vi "Get Control Values.vi"(8 "error in (no error)":errorcluster, 11 "Simulated Game Pad Interface in":refnum<class "Simulated Game Pad Interface.lvclass">) -> (0 "error out":errorcluster, 2 "Cluster":T1, 3 "Simulated Game Pad Interface out":refnum<class "Simulated Game Pad Interface.lvclass">)   [LabVIEW 2017, in "Simulated Game Pad Interface.lvclass"]
uses:
  Simulated Game Pad Interface.lvclass
  Abstract Game Pad Interface/Game Pad Descriptor.ctl
  Abstract Game Pad Interface/Abstract Game Pad Interface.lvclass
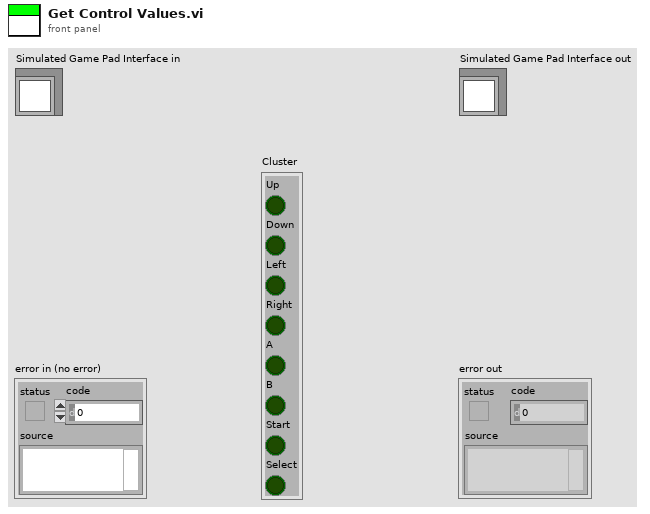
[diagram p1: front panel]
types:
  T1 = typedef "Abstract Game Pad Interface.lvclass/Game Pad Descriptor.ctl" = cluster{"Up":bool, "Down":bool, "Left":bool, "Right":bool, "A":bool, "B":bool, "Start":bool, "Select":bool}
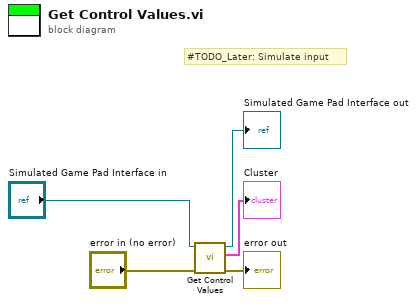
[diagram p0: block diagram]
diagram:
  # "#TODO_Later: Simulate input"
  n1 = call-parent "Get Control Values.vi"("error in (no error)"="error in (no error)", "Abstract Game Pad Interface in"="Simulated Game Pad Interface in") -> ("error out"=→"error out":errorcluster, "Cluster"=→"Cluster":T1, "Abstract Game Pad Interface out"=→"Simulated Game Pad Interface out":refnum<class "Simulated Game Pad Interface.lvclass">)  [unwired: 7 in]
